vi "WPI_DriverStationGetModeAndStatus.vi"() -> (2 "FMS Attached":bool, 3 "Robot Mode":T1)   [LabVIEW 2017]
doc: "This VI returns the mode and status of the robot. It tells if the robot in Teleop, Autonomous, Test, etc., and if the robot is connected to the FMS.\n\nThis software is licensed. Open the labview\\readme\\WPI Robotics Library Open Source License.txt file for more information."
uses:
  <vilib>/Rock Robotics/WPI/DriverStation/WPI_DriverStationRobotMode2.ctl
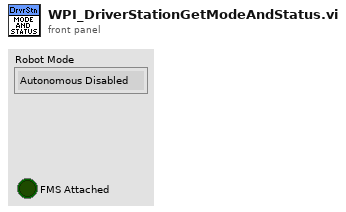
[diagram p1: front panel]
types:
  T1 = typedef "WPI_DriverStationRobotMode2.ctl" = enum16{"Autonomous Disabled", "Autonomous Enabled", "Teleop Disabled", "Teleop Enabled", "Disconnected", "Finish", "Test Disabled", "Test Enabled", "Emergency Stopped"}
  T2 = typedef "NetComm_ControlWord.ctl" = cluster{"Enabled":bool, "Autonomous":bool, "Test":bool, "E-Stop":bool, "FMS Attached":bool, "DS Attached":bool}
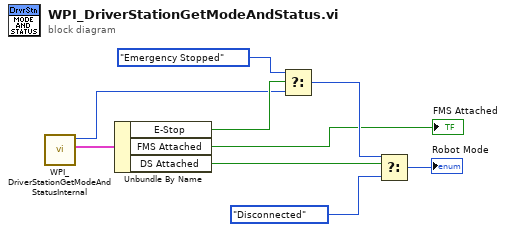
[diagram p0: block diagram]
diagram:
  n1 = call <vilib>:"WPI_DriverStationGetModeAndStatusInternal.vi"() -> ("Control Word"=w9:T2, "Robot Mode"=w4:T1)  [unwired: 10 in]
  n2 = Unbundle By Name(w9) -> ("E-Stop"=w8:bool, "FMS Attached"=→"FMS Attached":bool, "DS Attached"=w6:bool)
  n3 = Select(t=WPI_DriverStationRobotMode2."Emergency Stopped" ("Robot Mode"), s=w8, f=w4) -> (s? t:f=w3:T1)
  n4 = Select(t=w3, s=w6, f=WPI_DriverStationRobotMode2."Disconnected" ("Robot Mode")) -> (s? t:f=→"Robot Mode":T1)
